vi "DDS_client_event.vi"() -> ()   [LabVIEW 2012]
uses:
  <userlib>/LabRAD/internal/Build Packet SubVIs/Build Packet by Name.vi
  <userlib>/LabRAD/internal/Simple Request SubVIs/Simple Request by Name.vi
panel:
  in  "Amplitude (dBm)":dbl=-5.0 min=-63.0 max=-5.0 step=0.01 format="%_4g"
  in  "Frequency (MHz)":dbl=80.0 min=10.0 max=150.0 step=1e-09 format="%.9f"
  in  "Channel":u16(ring) items=["global397", "866DP"]
  out "client ID":u32
  out "welcome message":string
  in  "manager":T1={"address"="localhost", "port"=7682, "password"=""}
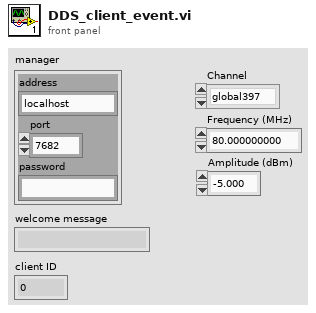
[diagram p1: front panel]
types:
  T1 = cluster{"address":string, "port":u16, "password":string}
  T2 = cluster{"RingText.Text":string, "Frequency (MHz)":dbl}
  T3 = cluster{"RingText.Text":string, "Amplitude (dBm)":dbl}
  T4 = cluster{"Setting":cluster{"ID":u32, "Name":string}, "Type Tag":string, "Data":string}[]
  T5 = cluster{"ID":u32, "Type Tag":string, "Data":string}[]
  T6 = cluster{"Setting":u32, "Type Tag":string, "Data":string}[]
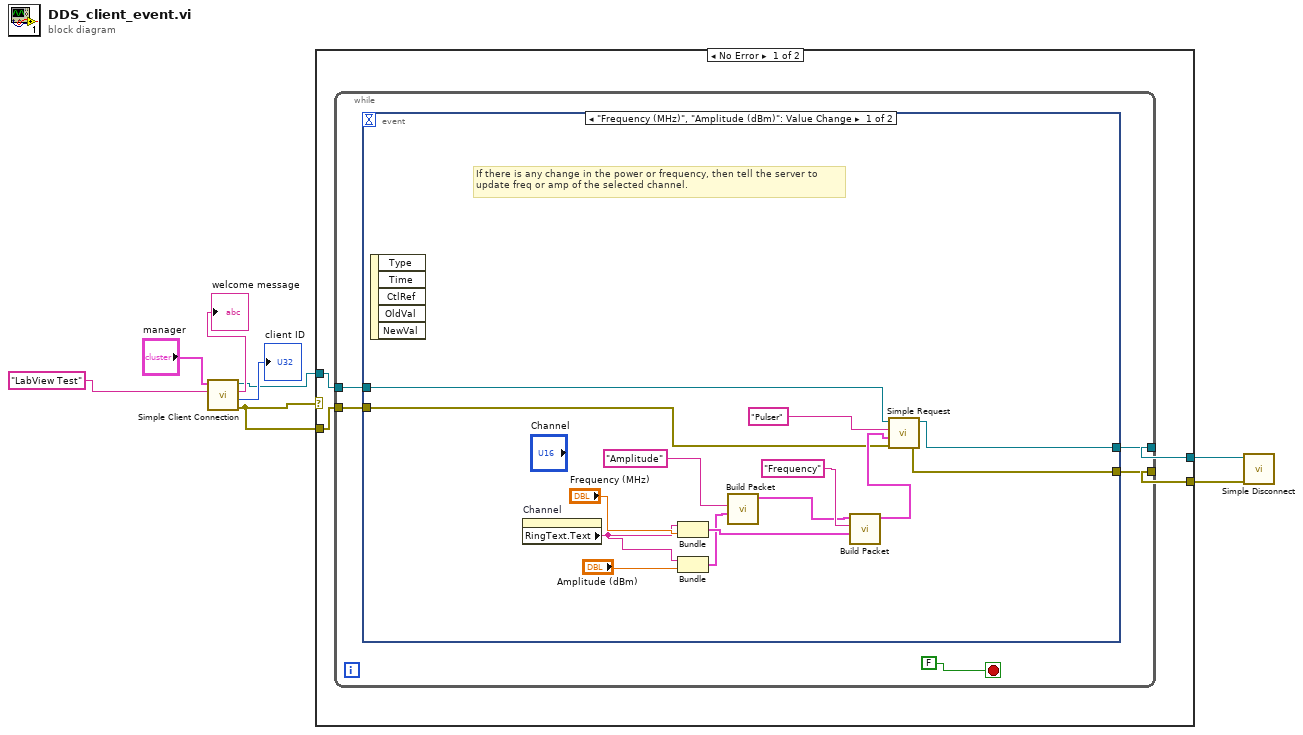
[diagram p0: block diagram]
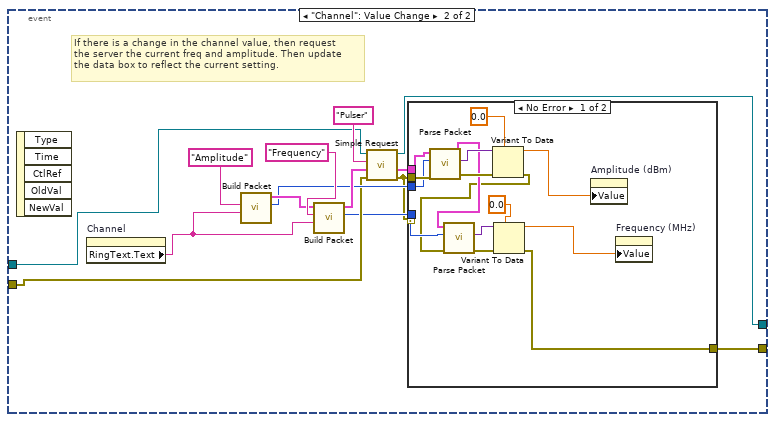
[diagram p2: hidden frame]
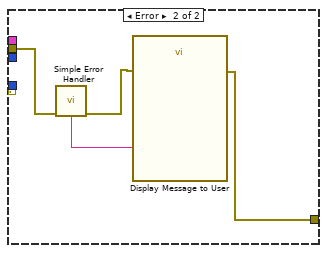
[diagram p3: hidden frame]
diagram:
  n1 = call <userlib>:"Simple Client Connection.vi"("connection name (LabVIEW Client)"="LabView Test", "manager"="manager") -> ("error out"=w1:errorcluster, "client ID"=→"client ID":u32, "welcome message"=→"welcome message":string, "connection ID out"=w4:refnum<k5>)  [unwired: 2 in]
  n2 = case shown="No Error" w1 {
    tunnel: w1 -> [w12 w65]
    tunnel: w4 -> [w11 w66]
    tunnel: [w10 w66] -> w3
    tunnel: [w9 w65] -> w2
    frame No Error {
      n3 = while {
        tunnel: w12 -> [w17]
        tunnel: w11 -> [w16]
        tunnel: [w15] -> w10
        tunnel: [w14] -> w9
        stop <- FALSE stop-if-true
        n4 = event shown="[0] \"Frequency (MHz)\", \"Amplitude (dBm)\": Value Change" {
          selector: _ -> [_ _]
          dyn-events: _ -> [_ _]
          timeout: _ -> [_ _]
          tunnel: w17 -> [w21 w38]
          tunnel: w16 -> [w20 w37]
          tunnel: [w19 w36] -> w15
          tunnel: [w18 w34] -> w14
          event "Frequency (MHz)", "Amplitude (dBm)": Value Change {
            # "If there is any change in the power or frequency, then tell the server to\nupdate freq or amp of the selected channel."
            n5 = event-data() -> ()  [unwired: 1 in, 5 out]
            n6 = property on="Channel" class="Ring (strict)"() -> ("RingText.Text"=w30:string)  [unwired: 2 in, 2 out]
            n7 = Bundle("RingText.Text"=w30, "Frequency (MHz)"="Frequency (MHz)") -> (w27:T2)  [unwired: 1 in]
            n8 = Bundle("RingText.Text"=w30, "Amplitude (dBm)"="Amplitude (dBm)") -> (w24:T3)  [unwired: 1 in]
            n9 = call-poly <userlib>:"Build Packet.vi"("data (empty)"=w24, "setting"="Amplitude") -> ("appended records"=w25:T4)  [unwired: 6 in, 2 out]
            n10 = call-poly <userlib>:"Build Packet.vi"("data (empty)"=w27, "setting"="Frequency", "records (empty)"=w25) -> ("appended records"=w26:T4)  [unwired: 5 in, 2 out]
            n11 = call-poly <userlib>:"Simple Request.vi"("error in (no error)"=w21, "records in (empty)"=w26, "target (Manager)"="Pulser", "connection ID"=w20) -> ("error out"=w18:errorcluster, "connection ID out"=w19:refnum<k5>)  [unwired: 2 in, 2 out]
          }
          event "Channel": Value Change {
            # "If there is a change in the channel value, then request\nthe server the current freq and amplitude. Then update\nthe data box to reflect the current setting."
            n12 = event-data() -> ()  [unwired: 1 in, 5 out]
            n13 = property on="Channel" class="Ring (strict)"() -> ("RingText.Text"=w33:string)  [unwired: 2 in, 2 out]
            n14 = call-poly <userlib>:"Build Packet.vi"("data (empty)"=w33, "setting"="Amplitude") -> ("index"=w39:u32, "appended records"=w43:T4)  [unwired: 6 in, 1 out]
            n15 = call-poly <userlib>:"Build Packet.vi"("data (empty)"=w33, "setting"="Frequency", "records (empty)"=w43) -> ("index"=w35:u32, "appended records"=w44:T4)  [unwired: 5 in, 1 out]
            n16 = call-poly <userlib>:"Simple Request.vi"("error in (no error)"=w38, "records in (empty)"=w44, "target (Manager)"="Pulser", "connection ID"=w37) -> ("error out"=w32:errorcluster, "records out"=w40:T5, "connection ID out"=w36:refnum<k5>)  [unwired: 2 in, 1 out]
            n17 = case shown="No Error" w32 {
              tunnel: w32 -> [w60 w63]
              tunnel: w40 -> [w59 _]
              tunnel: w39 -> [w58 _]
              tunnel: w35 -> [w53 _]
              tunnel: [w50 w64] -> w34
              frame No Error {
                n18 = call <userlib>:"Parse Packet.vi"("records"=w59, "index (0)"=w58, "error in (no error)"=w60) -> ("records out"=w54:T6, "data"=w57:variant, "error out"=w56:errorcluster)  [unwired: 3 in, 1 out]
                n19 = Variant To Data(error in=w56, type=0.0, Variant=w57) -> (data=w49:dbl, error out=w47:errorcluster)
                n20 = call <userlib>:"Parse Packet.vi"("records"=w54, "index (0)"=w53, "error in (no error)"=w47) -> ("data"=w52:variant, "error out"=w46:errorcluster)  [unwired: 3 in, 2 out]
                n21 = Variant To Data(error in=w46, type=0.0, Variant=w52) -> (data=w48:dbl, error out=w50:errorcluster)
                n22 = property on="Amplitude (dBm)" class="DigNum (strict)"("Value"=w49) -> ()  [unwired: 2 in, 2 out]
                n23 = property on="Frequency (MHz)" class="DigNum (strict)"("Value"=w48) -> ()  [unwired: 2 in, 2 out]
              }
              frame Error {
                n24 = call <vilib>:"Simple Error Handler.vi"("error in (no error)"=w63) -> ("error out"=w61:errorcluster, "message"=w62:string)  [unwired: 4 in, 3 out]
                n25 = call "Display Message to User"("error in (no error)"=w61, "Message"=w62) -> ("error out"=w64:errorcluster)  [unwired: 8 in, 1 out]
              }
            }
          }
        }
      }
    }
    frame Error {
    }
  }
  n26 = call <userlib>:"Simple Disconnect.vi"("error in (no error)"=w2, "connection ID"=w3) -> ()  [unwired: 5 in, 1 out]
